vi "Send Ref.vi"(8 "error in (no error)":errorcluster, 11 "Sync Box in":refnum<class "Sync Box.lvclass">) -> (0 "error out":errorcluster, 3 "Sync Box out":refnum<class "Sync Box.lvclass">)   [LabVIEW 2018, in "Sync Box.lvclass"]
uses:
  Sync Box.lvclass
  C:/Users/observer/Desktop/Sparc4GUI/SPARC4_GUI/Server/Server.lvclass
  Server/Server.lvclass/Server.ctl
  Server/Server.lvclass
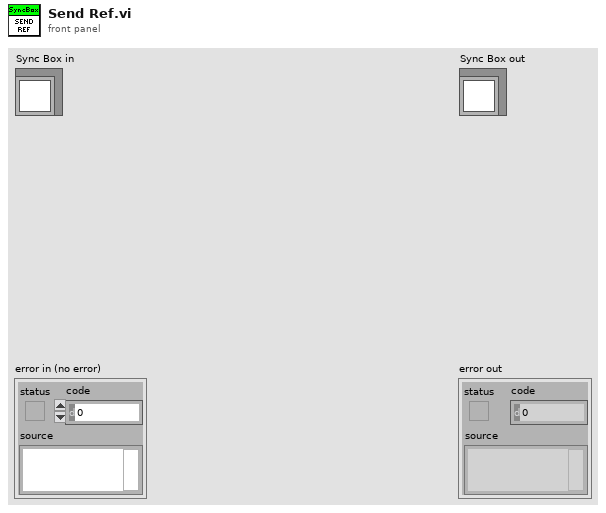
[diagram p1: front panel]
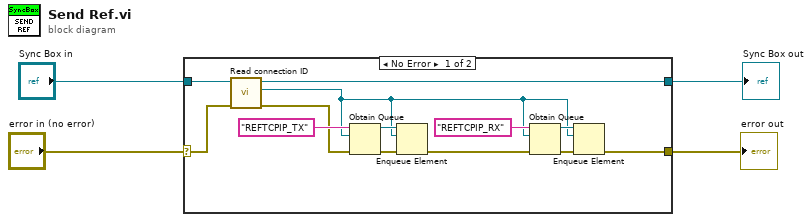
[diagram p0: block diagram]
diagram:
  n1 = case shown="No Error" "error in (no error)" {
    selector: "error in (no error)" -> [w8 w19]
    tunnel: [w10 w19] -> w2
    tunnel: [w7 w18] -> w1
    tunnel: "Sync Box in" -> [w9 w18]
    frame No Error {
      n2 = call "Read connection ID.vi"("error in (no error)"=w8, "Server in"=w9) -> ("error out"=w5:errorcluster, "connection ID"=w6:refnum<k5>, "Server out"=w7:refnum<class "Sync Box.lvclass">)  [unwired: 7 in]
      n3 = Obtain Queue(name (unnamed)="REFTCPIP_TX", element data type=w6, error in (no error)=w5) -> (queue out=w16:refnum<queue>, error out=w15:errorcluster)  [unwired: 2 in, 1 out]
      n4 = Enqueue Element(queue=w16, element=w6, error in (no error)=w15) -> (error out=w11:errorcluster)  [unwired: 1 in, 2 out]
      n5 = Obtain Queue(name (unnamed)="REFTCPIP_RX", element data type=w6, error in (no error)=w11) -> (queue out=w13:refnum<queue>, error out=w14:errorcluster)  [unwired: 2 in, 1 out]
      n6 = Enqueue Element(queue=w13, element=w6, error in (no error)=w14) -> (error out=w10:errorcluster)  [unwired: 1 in, 2 out]
    }
    frame Error {
    }
  }
  "error out" <- w2
  "Sync Box out" <- w1
